vi "Acq Configure Start Trigger.vi"(0 "session in":refnum<class "Digitizer Control.lvclass">, 1 "trigger type (Immediate)":T1, 3 "rising edge? (T)":bool=TRUE caption="rising edge?", 5 "error in (no error)":errorcluster, 6 "analog level (0)":dbl, 7 "digital trigger source (PXI_Trig0)":string(combo)="PXI_Trig0", 8 "analog hysteresis (0)":dbl, 9 "digital high level? (T)":bool=TRUE, 10 "analog trigger channel (AI0)":string="AI0") -> (14 "session out":refnum<class "Digitizer Control.lvclass">, 19 "error out":errorcluster)   [LabVIEW 2021, in "Digitizer Control.lvclass"]
doc: "Configures the acquisition start trigger. Use the <B>Acq Configure Channel.vi</B> to configure the channel parameters, and the <B>Acq Configure Transfer.vi</B> to configure the waveform transfer. Once the acquisition is configured, use the <B>Acq Initiate.vi</B> to initiate an acquisition, then use the <B>Acq Fetch Waveform.vi</B> to fetch the acquired samples. Use the <B>Acq Get Status.vi</B> to check the acquisition status and the <B>Acq Stop.vi</B> to stop an acquisition.\n\nInputs:\n\n<B>session in</B>: The device session.\n\n<B>trigger type</B>, <B>rising edge?</B>, <B>analog trigger channel</B>, <B>analog hysteresis</B>, <B>analog level</B>, <B>digital trigger source</B>, <B>digital high level?</B>: The <B>trigger type</B> input selects the start trigger type. If this input is \"Immediate\", then the acquisition triggers itself immediately and independently of external signals. If the <B>trigger type</B> input is \"Analog\", then the acquisition uses analog edge triggering. In this case use the <B>analog trigger channel</B> input to specify the channel to monitor for trigger conditions (AI0 or AI1), use the <B>rising edge?</B> input to specify whether to trigger on a rising or falling edge, use the <B>analog level</B> input to specify the trigger level in Volts, use the <B>analog hysteresis</B> input to specify the size of the hysteresis window on either side of <B>analog level</B> in Volts. If the <B>trigger type</B> input is \"Digital Edge\", then the acquisition uses digital edge triggering. In this case use the <B>digital trigger source</B> input to specify the trigger source and the <B>rising edge?</B> input to specify whether to trigger on a rising or falling edge. If the <B>trigger type</B> input is \"Digital Level\", then the acquisition triggers on a high or low level of a digital signal. In this case use the <B>digital trigger source</B> input to specify the trigger source and the <B>digital high level?</B> input to specify whether to trigger on a high or low level.\n\nOutputs:\n\n<B>session out</B>: The device session passed on the <B>session in</B> input."
uses:
  Digitizer Control.lvclass
  Acq Start Trigger Type.ctl
  Digitizer Control.lvclass/Digitizer Control.ctl
  <instrlib>/FlexRIO/API/Host/v1/NI FlexRIO/API/Configure Immediate Start Trigger.vi
  <instrlib>/FlexRIO/API/Host/v1/NI FlexRIO/API/Configure Analog Start Trigger.vi
  <instrlib>/FlexRIO/API/Host/v1/NI FlexRIO/API/Configure Digital Edge Start Trigger.vi
  <instrlib>/FlexRIO/API/Host/v1/NI FlexRIO/API/Configure Digital Level Start Trigger.vi
  <instrlib>/FlexRIO/API/Host/v1/NI FlexRIO API v1.lvlib
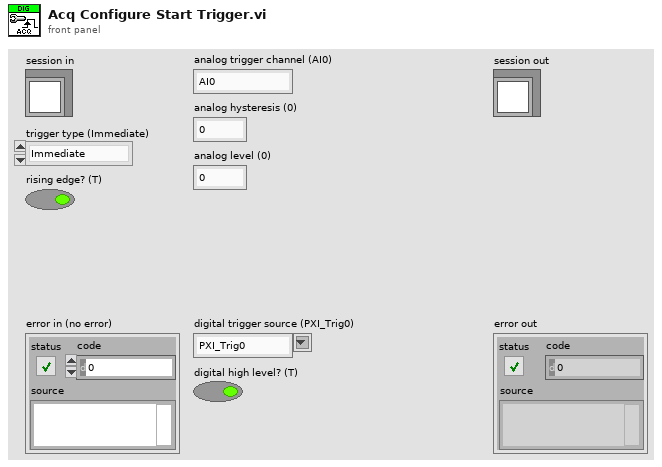
[diagram p1: front panel]
types:
  T1 = typedef "Digitizer Control.lvclass/Acq Start Trigger Type.ctl" = enum16{"Immediate", "Analog", "Digital Edge", "Digital Level"}
  T2 = typedef "Digitizer Control.lvclass/Acq Session Data.ctl" = cluster{"ADC sampling rate":dbl, "SCTL rate":dbl, "DMA element size (bits)":i32, "sample size (bits)":i32[], "DMA/memory interface width (DMA elements)":i32, "transfer size (bits)":i32[], "stream instance":i32[], "trigger instance":u32, "group delay (s)":dbl, "data delay (s)":dbl, "target delay (s)":dbl, "trigger tracking enabled":bool, "channel configured":bool, "enabled channels":bool[], "transfer configured":bool, "dsp bypass":bool, "fractional decimator input rate":dbl, "fractional decimator output rate":dbl, "sample scale factor":dbl[], "memory size":u64[], "FIFO size":u64}
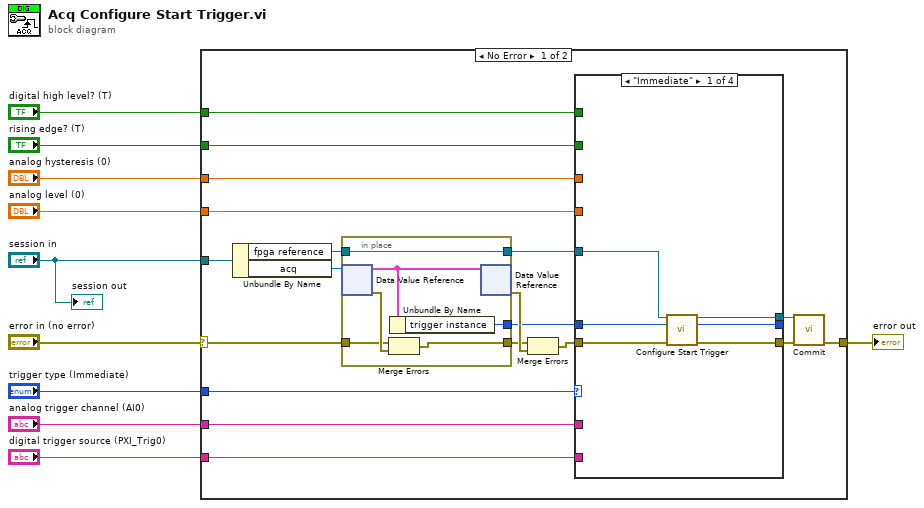
[diagram p0: block diagram]
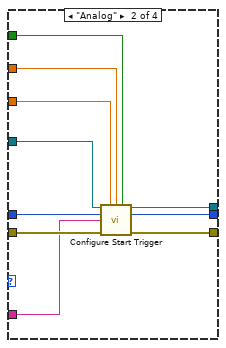
[diagram p2: hidden frame]
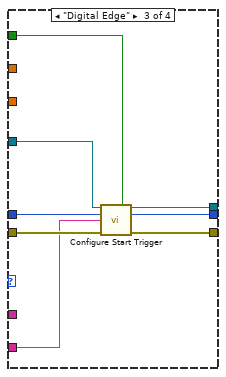
[diagram p3: hidden frame]
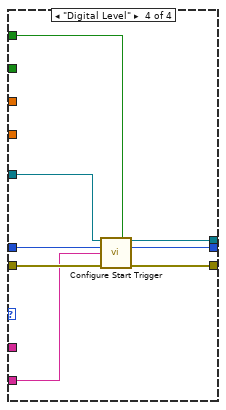
[diagram p4: hidden frame]
diagram:
  n1 = case shown="No Error" "error in (no error)" {
    selector: "error in (no error)" -> [w25 w68]
    tunnel: [w11 w68] -> w9
    tunnel: "session in" -> [w28 _]
    tunnel: "trigger type (Immediate)" -> [w20 _]
    tunnel: "analog level (0)" -> [w19 _]
    tunnel: "analog hysteresis (0)" -> [w18 _]
    tunnel: "rising edge? (T)" -> [w17 _]
    tunnel: "analog trigger channel (AI0)" -> [w16 _]
    tunnel: "digital trigger source (PXI_Trig0)" -> [w15 _]
    tunnel: "digital high level? (T)" -> [w14 _]
    frame No Error {
      n2 = Unbundle By Name(w28) -> ("fpga reference"=w27:refnum<k20>, "acq"=w26:refnum<data-value>)
      n3 = in-place {
        in-place-border: w27 -> [w64]
        in-place-border: w25 -> [w66]
        in-place-border: [w64] -> w24
        in-place-border: [w63] -> w22
        in-place-border: [w62] -> w23
        n4 = in-place-dvr #1(w26) -> (w65:T2, w67:errorcluster)
        n5 = Merge Errors(w66, w67) -> (w63:errorcluster)
        n6 = Unbundle By Name(w65) -> ("trigger instance"=w62:u32)
        n7 = in-place-dvr #1(w65) -> (w29:errorcluster)  [unwired: 1 out]
      }
      n8 = Merge Errors(w22, w29) -> (w21:errorcluster)
      n9 = case shown="\"Immediate\"" w20 {
        tunnel: w24 -> [w34 w44 w52 w60]
        tunnel: w23 -> [w33 w43 w51 w59]
        tunnel: w21 -> [w35 w45 w53 w61]
        tunnel: [w32 w42 w50 w58] -> w13
        tunnel: w19 -> [_ w41 _ _]
        tunnel: w18 -> [_ w40 _ _]
        tunnel: w17 -> [_ w39 w49 _]
        tunnel: w16 -> [_ w38 _ _]
        tunnel: w15 -> [_ _ w48 w57]
        tunnel: w14 -> [_ _ _ w56]
        tunnel: [w31 w37 w47 w55] -> w12
        tunnel: [w30 w36 w46 w54] -> _
        frame "Immediate" {
          n10 = call-poly <instrlib>:"Configure Start Trigger.vi"("fpga interface in"=w34, "trigger instance"=w33, "error in"=w35) -> ("fpga interface out"=w31:refnum<k20>, "trigger instance out"=w30:u32, "error out"=w32:errorcluster)  [unwired: 10 in]
        }
        frame "Analog" {
          n11 = call-poly <instrlib>:"Configure Start Trigger.vi"("fpga interface in"=w44, "level"=w41, "hysteresis"=w40, "rising edge?"=w39, "trigger instance"=w43, "channel"=w38, "error in"=w45) -> ("fpga interface out"=w37:refnum<k20>, "trigger instance out"=w36:u32, "error out"=w42:errorcluster)  [unwired: 6 in]
        }
        frame "Digital Edge" {
          n12 = call-poly <instrlib>:"Configure Start Trigger.vi"("fpga interface in"=w52, "rising edge?"=w49, "trigger instance"=w51, "trigger source"=w48, "error in"=w53) -> ("fpga interface out"=w47:refnum<k20>, "trigger instance out"=w46:u32, "error out"=w50:errorcluster)  [unwired: 8 in]
        }
        frame "Digital Level" {
          n13 = call-poly <instrlib>:"Configure Start Trigger.vi"("fpga interface in"=w60, "high level?"=w56, "trigger instance"=w59, "trigger source"=w57, "error in"=w61) -> ("fpga interface out"=w55:refnum<k20>, "trigger instance out"=w54:u32, "error out"=w58:errorcluster)  [unwired: 8 in]
        }
      }
      n14 = call <instrlib>:"Commit.vi"("fpga interface in"=w12, "error in"=w13) -> ("error out"=w11:errorcluster)  [unwired: 12 in, 1 out]
    }
    frame Error {
    }
  }
  "error out" <- w9
  "session out" <- "session in"
